vi "addDataU8Array.vi"(0 "U8ArrayBuilderAutoIndexing in":refnum<class "U8ArrayBuilderAutoIndexing.lvclass">, 5 "Data":u8[](array[numeric]), 7 "Length":i32, 11 "error in (no error)":errorcluster) -> (4 "U8ArrayBuilderAutoIndexing out":refnum<class "U8ArrayBuilderAutoIndexing.lvclass">, 15 "error out":errorcluster)   [LabVIEW 2016, in "RTUtilities.lvlib" / "U8ArrayBuilderAutoIndexing.lvclass"]
uses:
  U8ArrayBuilderAutoIndexing.lvclass
  U8ArrayBuilderAutoIndexing.lvclass/U8ArrayBuilderAutoIndexing.ctl
  U8ArrayBuilderManualIndexing/U8ArrayBuilderManualIndexing.lvclass
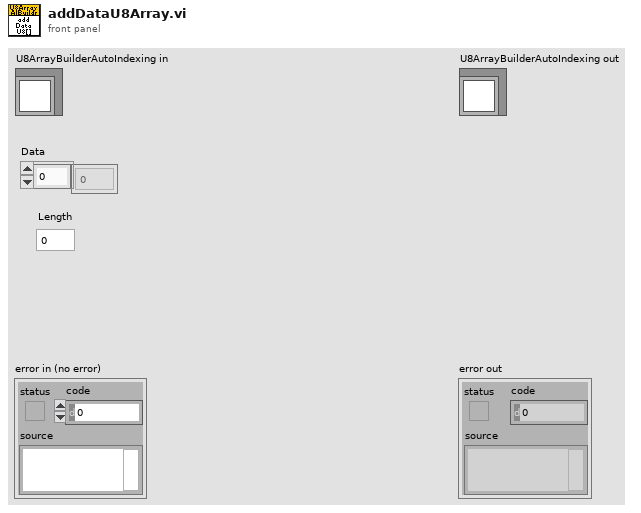
[diagram p1: front panel]
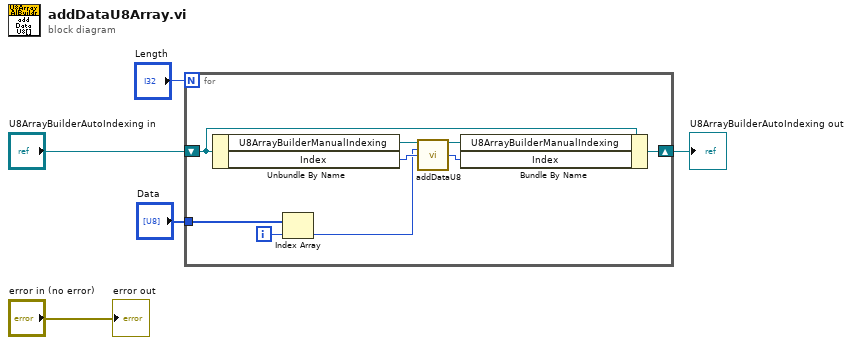
[diagram p0: block diagram]
diagram:
  n1 = for {
    N: "Length" -> [_]
    shift-right: [w9] -> w3
    shift-left: "U8ArrayBuilderAutoIndexing in" -> [w14]
    tunnel: "Data" -> [w8]
    i -> [w7]
    n2 = Unbundle By Name(w14) -> ("U8ArrayBuilderManualIndexing"=w13:refnum<class "U8ArrayBuilderManualIndexing.lvclass">, "Index"=w12:i32)
    n3 = Index Array(array=w8, index=w7) -> (element=w6:u8)
    n4 = call "addDataU8.vi"("U8ArrayBuilderManualIndexing in"=w13, "Data"=w6, "Index"=w12) -> ("U8ArrayBuilderManualIndexing out"=w10:refnum<class "U8ArrayBuilderManualIndexing.lvclass">, "Index out"=w11:i32)  [unwired: 10 in, 1 out]
    n5 = Bundle By Name(cluster=w14, "U8ArrayBuilderManualIndexing"=w10, "Index"=w11) -> (w9:refnum<class "U8ArrayBuilderAutoIndexing.lvclass">)
  }
  "U8ArrayBuilderAutoIndexing out" <- w3
  "error out" <- "error in (no error)"
